vi "Fix Offsets.vi"(4 "Rear Right":T1, 5 "Rear Left":T1, 6 "Front Left":T1, 7 "Front Right":T1) -> (0 "Rear Right":T1, 1 "Rear Left":T1, 2 "Front Left":T1, 3 "Front Right":T1)   [LabVIEW 2018]
uses:
  Final Motor Data.ctl
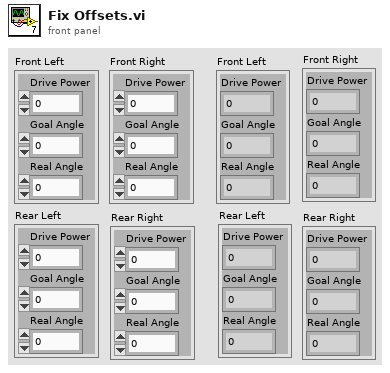
[diagram p1: front panel]
types:
  T1 = typedef "Final Motor Data.ctl" = cluster{"Drive Power":dbl, "Goal Angle":dbl, "Real Angle":dbl}
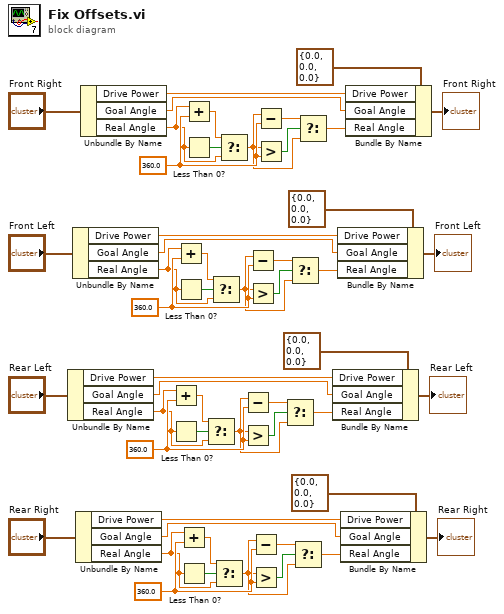
[diagram p0: block diagram]
diagram:
  w10 = 360.0
  w16 = 360.0
  w22 = 360.0
  w28 = 360.0
  n1 = Unbundle By Name("Rear Left") -> ("Drive Power"=w36:dbl, "Goal Angle"=w35:dbl, "Real Angle"=w2:dbl)
  n2 = Unbundle By Name("Front Left") -> ("Drive Power"=w38:dbl, "Goal Angle"=w37:dbl, "Real Angle"=w3:dbl)
  n3 = Unbundle By Name("Rear Right") -> ("Drive Power"=w34:dbl, "Goal Angle"=w33:dbl, "Real Angle"=w1:dbl)
  n4 = Unbundle By Name("Front Right") -> ("Drive Power"=w40:dbl, "Goal Angle"=w39:dbl, "Real Angle"=w4:dbl)
  n5 = Add(x=w2, y=w28) -> (x+y=w31:dbl)
  n6 = Less Than 0?(x=w2) -> (x < 0?=w32:bool)
  n7 = Add(x=w3, y=w16) -> (x+y=w19:dbl)
  n8 = Less Than 0?(x=w3) -> (x < 0?=w20:bool)
  n9 = Add(x=w1, y=w22) -> (x+y=w25:dbl)
  n10 = Less Than 0?(x=w1) -> (x < 0?=w26:bool)
  n11 = Add(x=w4, y=w10) -> (x+y=w13:dbl)
  n12 = Less Than 0?(x=w4) -> (x < 0?=w14:bool)
  n13 = Select(t=w31, s=w32, f=w2) -> (s? t:f=w27:dbl)
  n14 = Select(t=w19, s=w20, f=w3) -> (s? t:f=w15:dbl)
  n15 = Select(t=w25, s=w26, f=w1) -> (s? t:f=w21:dbl)
  n16 = Select(t=w13, s=w14, f=w4) -> (s? t:f=w9:dbl)
  n17 = Subtract(x=w27, y=w28) -> (x-y=w29:dbl)
  n18 = Greater?(x=w27, y=w28) -> (0:w30:bool)
  n19 = Subtract(x=w15, y=w16) -> (x-y=w17:dbl)
  n20 = Greater?(x=w15, y=w16) -> (0:w18:bool)
  n21 = Subtract(x=w21, y=w22) -> (x-y=w23:dbl)
  n22 = Greater?(x=w21, y=w22) -> (0:w24:bool)
  n23 = Subtract(x=w9, y=w10) -> (x-y=w11:dbl)
  n24 = Greater?(x=w9, y=w10) -> (0:w12:bool)
  n25 = Select(t=w29, s=w30, f=w27) -> (s? t:f=w6:dbl)
  n26 = Select(t=w17, s=w18, f=w15) -> (s? t:f=w7:dbl)
  n27 = Select(t=w23, s=w24, f=w21) -> (s? t:f=w5:dbl)
  n28 = Select(t=w11, s=w12, f=w9) -> (s? t:f=w8:dbl)
  n29 = Bundle By Name(cluster=T1 {"Drive Power"=0.0, "Goal Angle"=0.0, "Real Angle"=0.0} ("Front Right 2"), "Drive Power"=w36, "Goal Angle"=w35, "Real Angle"=w6) -> (→"Rear Left":T1)
  n30 = Bundle By Name(cluster=T1 {"Drive Power"=0.0, "Goal Angle"=0.0, "Real Angle"=0.0} ("Front Right 2"), "Drive Power"=w38, "Goal Angle"=w37, "Real Angle"=w7) -> (→"Front Left":T1)
  n31 = Bundle By Name(cluster=T1 {"Drive Power"=0.0, "Goal Angle"=0.0, "Real Angle"=0.0} ("Front Right 2"), "Drive Power"=w34, "Goal Angle"=w33, "Real Angle"=w5) -> (→"Rear Right":T1)
  n32 = Bundle By Name(cluster=T1 {"Drive Power"=0.0, "Goal Angle"=0.0, "Real Angle"=0.0} ("Front Right 2"), "Drive Power"=w40, "Goal Angle"=w39, "Real Angle"=w8) -> (→"Front Right":T1)
